vi "Custom PID.vi"(1 "Present Value":dbl format="%.3f", 2 "Set Point":dbl format="%.3g", 3 "Tuning Parameters":T1={"Controller Gain, Kc"=1.0, "Reset Time, Ti (s)"=0.01, "Derivative Time, Td (s)"=0.0} {"Derivative Time, Td (s)" format="%.3g"; "Reset Time, Ti (s)" format="%.3g"; "Controller Gain, Kc" format="%.3g"}) -> (0 "Controller Output":dbl format="%.3g")   [LabVIEW 2012]
panel:
  out "dt (min)":dbl format="%.3g"
  in  "dT (s)":dbl=-1.0 step=0.001 format="%.3f"
  # "This PID VI is meant to be used for instructional Purposes.  It is in ideal form and simplified down from the orginal PID VI from the default NI PID VI."
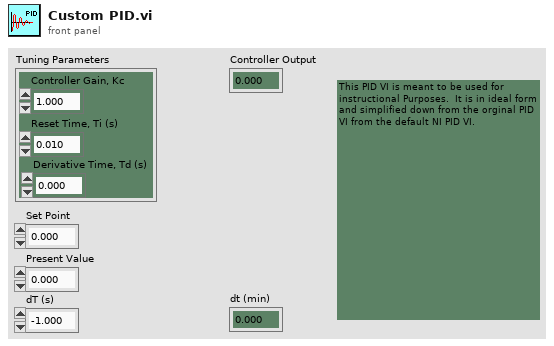
[diagram p1: front panel]
types:
  T1 = cluster{"Controller Gain, Kc":dbl, "Reset Time, Ti (s)":dbl, "Derivative Time, Td (s)":dbl}
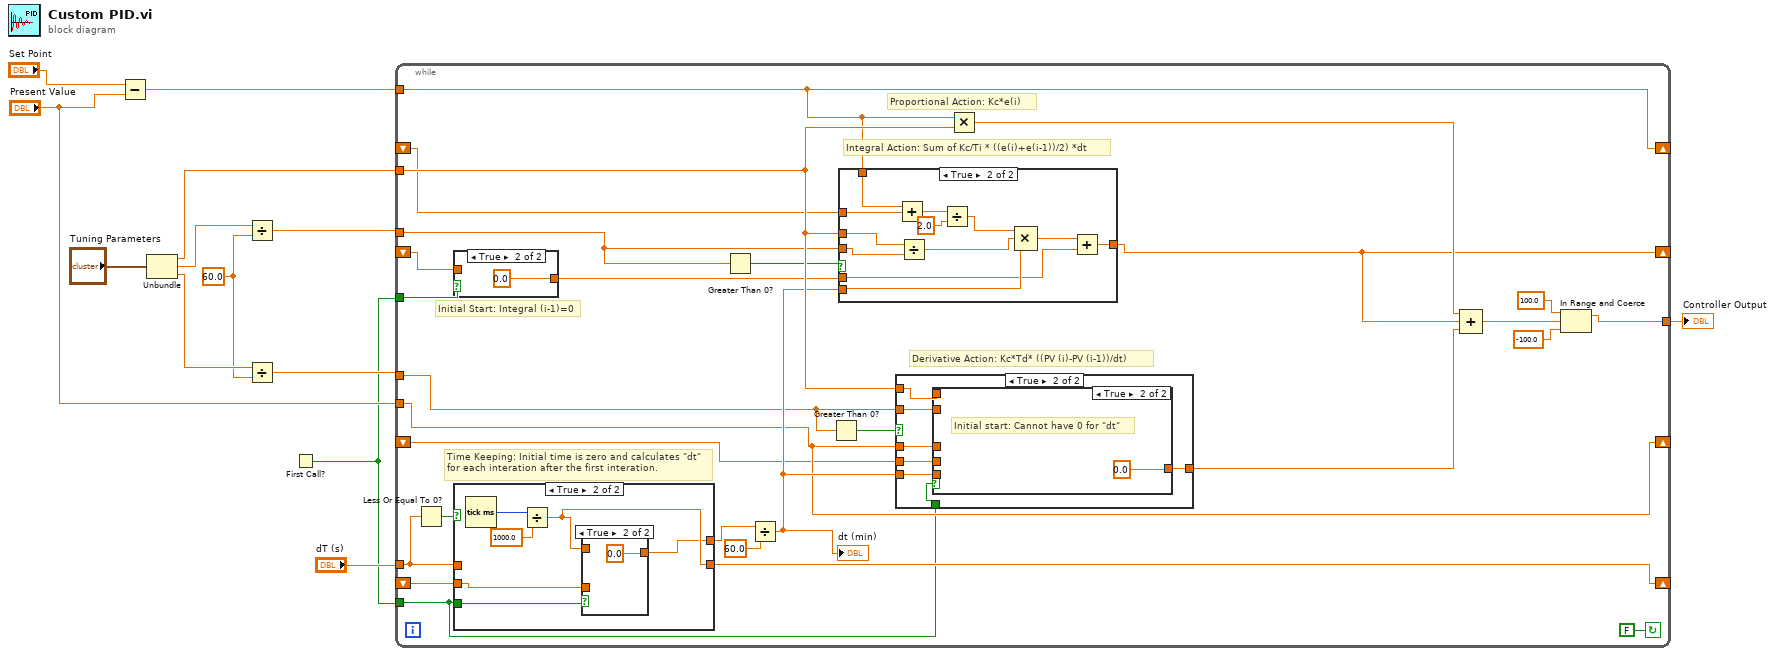
[diagram p0: block diagram]
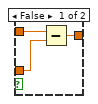
[diagram p4: hidden frame]
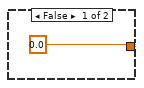
[diagram p5: hidden frame]
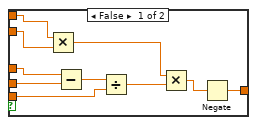
[diagram p6: hidden frame]
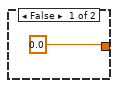
[diagram p7: hidden frame]
diagram:
  w4 = 60.0
  n1 = Subtract(x="Set Point", y="Present Value") -> (x-y=w12:dbl)
  n2 = Unbundle("Tuning Parameters") -> ("Controller Gain, Kc"=w8:dbl, "Reset Time, Ti (s)"=w10:dbl, "Derivative Time, Td (s)"=w9:dbl)
  n3 = Divide(x=w10, y=w4) -> (x/y=w7:dbl)
  n4 = Divide(x=w9, y=w4) -> (x/y=w6:dbl)
  n5 = First Call?() -> (First Call?: T/F=w1:bool)
  n6 = while {
    tunnel: w12 -> [w39]
    tunnel: w8 -> [w41]
    tunnel: w7 -> [w34]
    tunnel: w6 -> [w19]
    shift-right: [w39] -> _
    shift-left: _ -> [w40]
    tunnel: w1 -> [w17]
    shift-right: [w27] -> _
    shift-left: _ -> [w38]
    tunnel: "dT (s)" -> [w36]
    shift-right: [w29] -> _
    shift-left: _ -> [w15]
    tunnel: "Present Value" -> [w32]
    shift-right: [w32] -> _
    shift-left: _ -> [w31]
    tunnel: [w21] -> w2
    tunnel: w1 -> [w16]
    stop <- FALSE continue-if-true
    # "Initial Start: Integral (i-1)=0"
    # "Derivative Action: Kc*Td* ((PV (i)-PV (i-1))/dt)"
    # "Proportional Action: Kc*e(i)"
    # "Integral Action: Sum of Kc/Ti * ((e(i)+e(i-1))/2) *dt"
    # "Time Keeping: Initial time is zero and calculates \"dt\" for each interation after the first interation."
    n7 = Less Or Equal To 0?(x=w36) -> (x <= 0?=w37:bool)
    n8 = case shown="True" w16 {
      tunnel: w15 -> [w42 _]
      tunnel: [w42 0.0] -> w14
      frame False {
      }
      frame True {
      }
    }
    n9 = case shown="True" w37 {
      tunnel: w17 -> [_ w50]
      tunnel: [w44 w47] -> w27
      tunnel: w38 -> [_ w48]
      tunnel: w36 -> [w44 _]
      tunnel: [w44 w45] -> w26
      frame False {
      }
      frame True {
        n10 = Tick Count (ms)() -> (millisecond timer value=w49:u32)
        n11 = Divide(x=w49, y=1000.0) -> (x/y=w47:dbl)
        n12 = case shown="True" w50 {
          tunnel: w47 -> [w53 _]
          tunnel: w48 -> [w52 _]
          tunnel: [w51 0.0] -> w45
          frame False {
            n13 = Subtract(x=w53, y=w52) -> (x-y=w51:dbl)
          }
          frame True {
          }
        }
      }
    }
    n14 = Greater Than 0?(x=w34) -> (x > 0?=w33:bool)
    n15 = Divide(x=w26, y=60.0) -> (x/y=w35:dbl)
    "dt (min)" <- w35
    n16 = Greater Than 0?(x=w19) -> (x > 0?=w20:bool)
    n17 = case shown="True" w33 {
      tunnel: w41 -> [_ w82]
      tunnel: w34 -> [_ w81]
      tunnel: w40 -> [_ w83]
      tunnel: w39 -> [_ w84]
      tunnel: w35 -> [_ w78]
      tunnel: [0.0 w76] -> w29
      tunnel: w14 -> [_ w75]
      frame False {
      }
      frame True {
        n18 = Add(x=w84, y=w83) -> (x+y=w86:dbl)
        n19 = Divide(x=w82, y=w81) -> (x/y=w79:dbl)
        n20 = Divide(x=w86, y=2.0) -> (x/y=w80:dbl)
        n21 = Compound Arithmetic op=MULTIPLY(w80, w79, w78) -> (w77:dbl)
        n22 = Add(x=w77, y=w75) -> (x+y=w76:dbl)
      }
    }
    n23 = case shown="True" w20 {
      tunnel: w41 -> [_ w59]
      tunnel: w19 -> [_ w58]
      tunnel: w35 -> [_ w60]
      tunnel: w32 -> [_ w62]
      tunnel: w31 -> [_ w61]
      tunnel: [0.0 w57] -> w28
      tunnel: w17 -> [_ w56]
      frame False {
      }
      frame True {
        n24 = case shown="True" w56 {
          tunnel: w62 -> [w72 _]
          tunnel: w61 -> [w71 _]
          tunnel: w60 -> [w69 _]
          tunnel: w59 -> [w68 _]
          tunnel: w58 -> [w67 _]
          tunnel: [w63 0.0] -> w57
          frame False {
            n25 = Multiply(x=w68, y=w67) -> (x*y=w66:dbl)
            n26 = Subtract(x=w72, y=w71) -> (x-y=w70:dbl)
            n27 = Divide(x=w70, y=w69) -> (x/y=w65:dbl)
            n28 = Multiply(x=w66, y=w65) -> (x*y=w64:dbl)
            n29 = Negate(x=w64) -> (-x=w63:dbl)
          }
          frame True {
            # "Initial start: Cannot have 0 for \"dt\""
          }
        }
      }
    }
    n30 = Multiply(x=w39, y=w41) -> (x*y=w30:dbl)
    n31 = Compound Arithmetic op=ADD(w30, w29, w28) -> (w22:dbl)
    n32 = In Range and Coerce(upper limit=100.0 ("x"), x=w22, lower limit=-100.0 ("x")) -> (coerced(x)=w21:dbl)  [unwired: 1 out]
  }
  "Controller Output" <- w2
